vi "TEST_ASIC_MAJnADDS_NEW.vi"(0 "Instrument VISA in":T1={"AWG VISA"="generadorpulsos", "Oscilloscope  VISA "="Oscilloscope", "Integration Board IP"="172.16.7.43", "connection ID"=refnum, "report out"=refnum, "report file path"=path "C:/Documents and Settings/CTA_LAB01/Desktop/L0_Asic/L0 Asic Test Data"}, 1 "threshold":i32[][](array[numeric])=[[518, 513, 533, 498, 543, 508, 548], [526, 521, 546, 506, 551, 516, 556], [534, 529, 549, 514, 559, 524, 564], [542, 537, 557, 522, 567, 532, 572], [545, 540, 565, 530, 575, 530, 575]], 2 "Serial number":string="SN_023", 11 "error in":errorcluster, 13 "Voltages comprobation":dbl[](array[numeric])=[0.05, 0.1, 0.2, 0.5, 0.8]) -> (4 "Instrument VISA out":T1={"AWG VISA"="generadorpulsos", "Oscilloscope  VISA "="Oscilloscope", "Integration Board IP"="172.16.7.43", "connection ID"=refnum, "report out"=refnum, "report file path"=path "C:/Documents and Settings/CTA_LAB01/Desktop/L0_Asic/L0 Asic Test Data"}, 15 "error out":errorcluster)   [LabVIEW 2012]
uses:
  <vilib>/Utility/NIReport.llb/NI_report.lvclass
  Sum_Abrilader/L0_Sum_Adder Folder/C/Program Files/National Instruments/LabVIEW 2012/instr.lib/Agilent 81150/Agilent 81150.lvlib
  <instrlib>/Agilent 8000 Series/Agilent 8000 Series.lvlib
panel:
  in  "Attenuation":i32=15
  in  "NChannels":i32[](array[numeric])=[2, 2, 2, 2, 3, 3, 3, 4, 4, 5, 5, 6, 6, 7]
  in  "Channels Combinations":i32[](array[numeric])=[3, 12, 48, 96, 7, 28, 112, 15, 120, 31, 124, 63, 126, 127]
  out "read buffer 4":string="-1.1741E-08;2.232E-09;9.99999E+37;2.976E-09;3.8996E-01;3.7534E-01\n"
  out "ouput data array":dbl[](array[numeric])=[0.2, 127.0, 0.0, 564.0, 0.0, 0.7653, 0.0, 2.976e-09, 0.0, 9.99999e+37, 0.0, 2.232e-09, 0.0, -1.1741e-08, 0.0, 0.0]
  out "read buffer 3":string="V amptd(f2),1.074E+00,0,1.056E+00,1.087E+00,1.0690E+00,5.5E-03,9.4E+01,+ width(f2),2.90015E-09,0,2.90015E-09,2.95960E-09,2.925838E-09,1.2702E-11,9.4E+01,V amptd(1),5.5E-02,0,4.8E-02,6.7E-02,5.55E-02,3.5E-03,9.4E+01,+ width(f1),9.99999E+37,5,9.99999E+37,9.99999E+37,9.99999E+37,9.99999E+37,9.99999E+37,Time(f1-f2),6.26722E-09,0,6.20145E-09,6.35270E-09,6.264189E-09,3.2805E-11,9.4E+01\n"
  in  "Input Voltages":dbl[](array[numeric])=[0.05, 0.2]
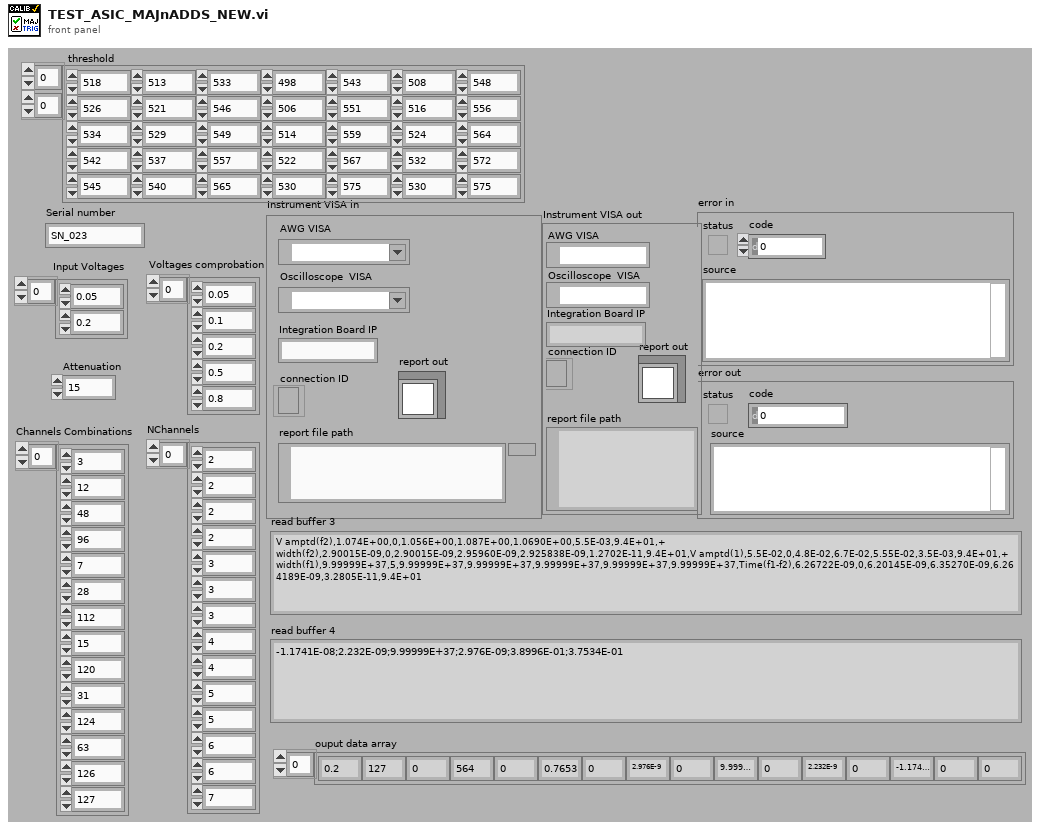
[diagram p1: front panel]
types:
  T1 = cluster{"AWG VISA":refnum<visa-resource-name>, "Oscilloscope  VISA ":refnum<visa-resource-name>, "Integration Board IP":string, "connection ID":refnum<k5>, "report out":refnum<class "NI_report.lvclass">, "report file path":path}
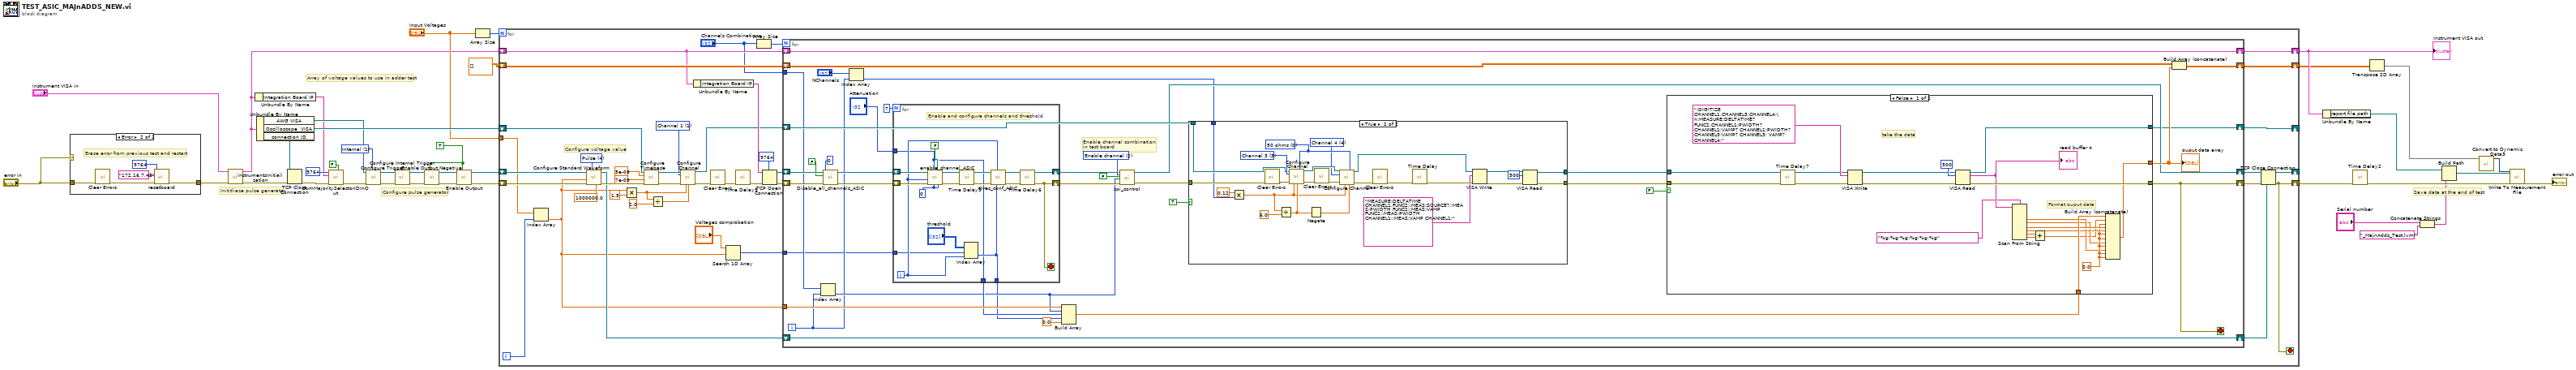
[diagram p0: block diagram]
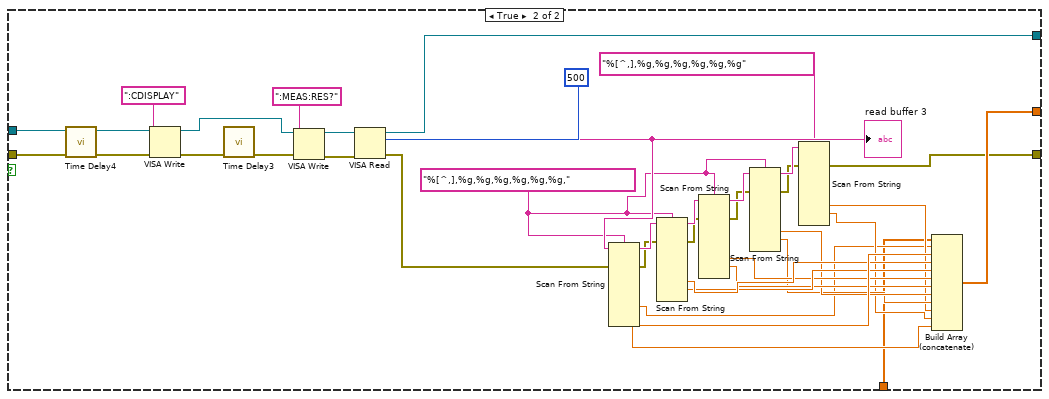
[diagram p3: hidden frame]
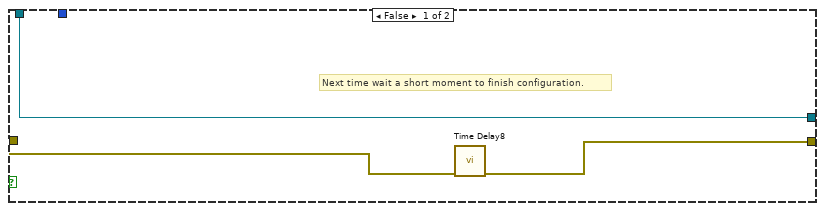
[diagram p4: hidden frame]
diagram:
  w24 = u16 1 items=["Immediate", "Internal", "External", "Software Trigger Function"] ("Trigger Source (0: Immediate)")
  w13 = TRUE ("Enable Output (T: Enable)")
  # "Save data at the end of test"
  # "Array of voltage values to use in adder test"
  # "Configure pulse generator"
  # "Inititliaze pulse generator"
  n1 = case shown="Error" "error in" {
    tunnel: "error in" -> [w39 w41]
    tunnel: [w39 w44] -> w21
    frame No Error {
    }
    frame Error {
      # "Erase error from previous test and restart"
      n2 = call <vilib>:"Clear Errors.vi"("error in (no error)"=w41) -> ("error out"=w40:errorcluster)  [unwired: 6 in]
      n3 = call "resetboard.vi"("error in (no error)"=w40, "address"="172.16.7.43", "remote port or service name"=u16 9764) -> ("error out"=w44:errorcluster)  [unwired: 7 in, 1 out]
    }
  }
  n4 = call "instrumentsInitialization.vi"("error in"=w21, "Instrument VISA in"="Instrument VISA in") -> ("error out"=w19:errorcluster, "Instrument VISA out"=w8:T1)  [unwired: 8 in]
  n5 = Unbundle By Name(w8) -> ("Integration Board IP"=w3:string)
  n6 = Unbundle By Name(w8) -> ("AWG VISA"=w27:refnum<visa-resource-name>, "Oscilloscope  VISA"=w33:refnum<visa-resource-name>, "connection ID"=w20:refnum<k5>)
  n7 = TCP Close Connection(connection ID=w20, error in (no error)=w19) -> (error out=w7:errorcluster)  [unwired: 1 in, 1 out]
  n8 = call "SumMajoritySelectorIDInOut.vi"("On Sum\nOff Majority"=FALSE ("Enable Output (T: Enable)"), "error in"=w7, "address"=w3, "remote port or service name"=u16 9764) -> ("error out"=w6:errorcluster)  [unwired: 7 in]
  n9 = call <instrlib>:"Configure Trigger.vi"("Trigger Source (0: Immediate)"=w24, "error in (no error)"=w6, "VISA resource name"=w27) -> ("error out"=w25:errorcluster, "VISA resource name out"=w26:refnum<visa-resource-name>)  [unwired: 7 in]
  n10 = call <instrlib>:"Configure Internal Trigger.vi"("error in (no error)"=w25, "VISA resource name"=w26) -> ("error out"=w15:errorcluster, "VISA resource name out"=w16:refnum<visa-resource-name>)  [unwired: 8 in]
  n11 = call "Enable Output Negative.vi"("Enable Output (T: Enable)"=w13, "error in (no error)"=w15, "VISA resource name"=w16) -> ("error out"=w14:errorcluster, "VISA resource name out"=w17:refnum<visa-resource-name>)  [unwired: 7 in]
  n12 = call <instrlib>:"Enable Output.vi"("Enable Output (T: Enable)"=w13, "error in (no error)"=w14, "VISA resource name"=w17) -> ("error out"=w2:errorcluster, "VISA resource name out"=w38:refnum<visa-resource-name>)  [unwired: 7 in]
  n13 = Array Size(array="Input Voltages") -> (size(s)=w34:i32)
  n14 = for {
    N: w34 -> [_]
    shift-right: [w75] -> w28
    shift-left: w2 -> [w84]
    tunnel: "Input Voltages" -> [w82]
    shift-right: [w79] -> w18
    shift-left: w8 -> [w52]
    shift-right: [w78] -> w12
    shift-left: dbl[][] [] -> [w80]
    shift-right: [w76] -> _
    shift-left: w38 -> [w83]
    shift-right: [w77] -> _
    shift-left: w33 -> [w81]
    i -> [w46]
    stop <- w75 stop-if-true
    w66 = 1 items=["Channel 1"=1, "Channel 2"=2, "Channel 3"=3, "Channel 4"=4] ("Channel (1: Channel 1)")
    w74 = u16 4 items=["Sine", "Square", "Ramp Up", "Ramp Down", "Pulse", "Noise", "DC"] ("Waveform (0: Sine)")
    # "Configure voltage value"
    n15 = Index Array(array=w82, index=w46) -> (element=w47:dbl)
    n16 = call <instrlib>:"Configure Standard Waveform.vi"("Frequency (1000.0 Hz)"=1000000.0, "Waveform (0: Sine)"=w74, "error in (no error)"=w84, "Amplitude (1.0 Vpp)"=w47, "VISA resource name"=w83) -> ("error out"=w72:errorcluster, "VISA resource name out"=w55:refnum<visa-resource-name>)  [unwired: 5 in]
    n17 = Multiply(x=w47, y=1.5) -> (x*y=w50:dbl)
    n18 = call <instrlib>:"Configure Timebase.vi"("error in (no error)"=w72, "Position (0.0 s)"=7e-09, "Timebase (0.005 s)"=5e-08, "VISA resource name"=w81) -> ("error out"=w71:errorcluster, "VISA resource name out"=w69:refnum<visa-resource-name>)  [unwired: 6 in]
    n19 = Divide(x=w50, y=2.0) -> (x/y=w60:dbl)
    n20 = call <instrlib>:"Configure Channel.vi"("VISA resource name"=w69, "Channel (1: Channel 1)"=w66, "error in (no error)"=w71, "Vertical Range (2.0 V)"=w50, "Vertical Offset (0.0 V)"=w60) -> ("VISA resource name out"=w59:refnum<visa-resource-name>, "error out"=w70:errorcluster)  [unwired: 9 in]
    n21 = Unbundle By Name(w52) -> ("Integration Board IP"=w63:string)
    n22 = call <vilib>:"Clear Errors.vi"("error in (no error)"=w70) -> ("error out"=w54:errorcluster)  [unwired: 6 in]
    n23 = Search 1D Array(1D array="Voltages comprobation", element=w47) -> (index of element=w45:i32)  [unwired: 1 in]
    n24 = call "Time Delay5"("error in (no error)"=w54) -> ("error out"=w53:errorcluster)  [unwired: 10 in]
    n25 = Array Size(array="Channels Combinations") -> (size(s)=w49:i32)
    n26 = TCP Open Connection(address=w63, remote port or service name=u16 9764, error in (no error)=w53) -> (connection ID=w56:refnum<k5>, error out=w64:errorcluster)  [unwired: 2 in]
    n27 = for {
      N: w49 -> [_]
      shift-right: [w106] -> w58
      shift-left: w64 -> [w116]
      shift-right: [w117] -> w78
      shift-left: w80 -> [w118]
      shift-right: [w107] -> w57
      shift-left: w56 -> [w105]
      tunnel: w47 -> [w104]
      shift-right: [w101] -> w77
      shift-left: w59 -> [w110]
      shift-right: [w100] -> w76
      shift-left: w55 -> [w100]
      shift-right: [w96] -> w79
      shift-left: w52 -> [w96]
      tunnel: "Channels Combinations" -> [w93]
      tunnel: w45 -> [w86]
      i -> [w89]
      stop <- w106 stop-if-true
      w115 = u16 2 items=["Attenuation", "Clipping", "Enable channel", "Delay line", "ASIC"] ("Device")
      # "Enable channel combination \nin test board"
      n28 = Index Array(array=w93, index=w89) -> (element=w92:i32)
      n29 = call "Disable_all_channels_ASIC.vi"("error in"=w116, "id_in"=0 ("Data"), "Clip_en_b"=FALSE, "connection ID"=w105) -> ("error out"=w120:errorcluster, "connection ID out"=w119:refnum<k5>)  [unwired: 5 in, 1 out]
      n30 = Index Array(array="NChannels", index=w89) -> (element=w88:i32)
      n31 = for {
        N: u32 7 ("Att gain") -> [_]
        shift-right: [w217] -> w113
        shift-left: w120 -> [w223]
        shift-right: [w218] -> w112
        shift-left: w119 -> [w222]
        tunnel: [w209] -> w103
        tunnel: [w212] -> w91
        tunnel: w86 -> [w210]
        tunnel: "Attenuation" -> [w209]
        i -> [w211]
        stop <- w217 stop-if-true
        w220 = u32 0 ("Ib_clipVb")
        # "Enable and configure channels and threshold"
        n32 = call "enable_channel_ASIC.vi"("Clip_sel_b"=w220, "maj/sum"=FALSE, "Ib_clipVb"=w220, "Att gain"=w209, "error in"=w223, "Channel"=w211, "connection ID"=w222) -> ("error out"=w214:errorcluster, "connection ID out"=w219:refnum<k5>)  [unwired: 2 in, 1 out]
        n33 = call "Time Delay9"("error in (no error)"=w214) -> ("error out"=w215:errorcluster)  [unwired: 10 in]
        n34 = Index Array(array="threshold", index (row)=w210, index (col)=w211) -> (element=w212:i32)
        n35 = call "thres_conf_ASIC.vi"("threshold"=w212, "Ring"=w211, "error out 3"=w215, "connection ID"=w219) -> ("error out 2"=w216:errorcluster, "connection ID out"=w218:refnum<k5>)  [unwired: 4 in, 2 out]
        n36 = call "Time Delay6"("error in (no error)"=w216) -> ("error out"=w217:errorcluster)  [unwired: 10 in]
      }
      n37 = Build Array(w104, w92, w103, w91, 0.0 ("element")) -> (w102:dbl[])
      n38 = call "spi_control.vi"("connection ID"=w112, "Device"=w115, "Read/#write"=FALSE, "Data"=w92, "error out 3"=w113) -> ("connection ID out"=w107:refnum<k5>, "error out 2"=w111:errorcluster)  [unwired: 7 in, 6 out]
      n39 = case shown="True" TRUE {
        tunnel: [w181 w194] -> w98
        tunnel: w111 -> [w182 w189]
        tunnel: w110 -> [w183 w190]
        tunnel: [w183 w200] -> w109
        tunnel: w88 -> [_ w185]
        frame False {
          # "Next time wait a short moment to finish configuration."
          n40 = call "Time Delay8"("error in (no error)"=w182) -> ("error out"=w181:errorcluster)  [unwired: 10 in]
        }
        frame True {
          w201 = u32 0 items=["50 ohms", "1 Mohms"] ("Input Impedance (1: 1 Mohms)")
          w193 = 3 items=["Channel 1"=1, "Channel 2"=2, "Channel 3"=3, "Channel 4"=4] ("Channel (1: Channel 1)")
          w192 = 4 items=["Channel 1"=1, "Channel 2"=2, "Channel 3"=3, "Channel 4"=4] ("Channel (1: Channel 1)")
          n41 = Multiply(x=0.12 ("y"), y=w185) -> (x*y=w186:dbl)
          n42 = call <vilib>:"Clear Errors.vi"("error in (no error)"=w189) -> ("error out"=w207:errorcluster)  [unwired: 6 in]
          n43 = Divide(x=w186, y=6.0) -> (x/y=w187:dbl)
          n44 = call <instrlib>:"Configure Channel.vi"("VISA resource name"=w190, "Input Impedance (1: 1 Mohms)"=w201, "Channel (1: Channel 1)"=w193, "error in (no error)"=w207, "Vertical Range (2.0 V)"=w186, "Vertical Offset (0.0 V)"=w187) -> ("VISA resource name out"=w205:refnum<visa-resource-name>, "error out"=w208:errorcluster)  [unwired: 8 in]
          n45 = Negate(x=w187) -> (-x=w191:dbl)
          n46 = call <vilib>:"Clear Errors.vi"("error in (no error)"=w208) -> ("error out"=w199:errorcluster)  [unwired: 6 in]
          n47 = call <instrlib>:"Configure Channel.vi"("VISA resource name"=w205, "Input Impedance (1: 1 Mohms)"=w201, "Channel (1: Channel 1)"=w192, "error in (no error)"=w199, "Vertical Range (2.0 V)"=w186, "Vertical Offset (0.0 V)"=w191) -> ("VISA resource name out"=w197:refnum<visa-resource-name>, "error out"=w206:errorcluster)  [unwired: 8 in]
          n48 = call <vilib>:"Clear Errors.vi"("error in (no error)"=w206) -> ("error out"=w198:errorcluster)  [unwired: 6 in]
          n49 = call "Time Delay"("error in (no error)"=w198) -> ("error out"=w196:errorcluster)  [unwired: 10 in]
          n50 = VISA Write(VISA resource name=w197, write buffer="MEASURE:DELTATIME CHANNEL1,FUNC2;:MEAS:SOURCE?;:MEAS:PWIDTH FUNC2;:MEAS:VAMP FUNC2;:MEAS:PWIDTH CHANNEL1;:MEAS:VAMP CHANNEL1;", error in (no error)=w196) -> (VISA resource name out=w204:refnum<visa-resource-name>, error out=w203:errorcluster)  [unwired: 1 out]
          n51 = VISA Read(VISA resource name=w204, byte count=u32 500, error in (no error)=w203) -> (VISA resource name out=w200:refnum<visa-resource-name>, error out=w194:errorcluster)  [unwired: 2 out]
        }
      }
      n52 = case shown="False" FALSE {
        tunnel: w109 -> [w139 w151]
        tunnel: [w134 w149] -> w108
        tunnel: [w137 w148] -> w106
        tunnel: w102 -> [w135 w146]
        tunnel: [w136 w145] -> w101
        tunnel: w98 -> [w138 w143]
        frame False {
          w130 = 0.0 ("output 7")
          # "Format ouput data"
          # "take the data"
          n53 = call "Time Delay7"("error in (no error)"=w138) -> ("error out"=w140:errorcluster)  [unwired: 10 in]
          n54 = VISA Write(VISA resource name=w139, write buffer=":DIGITIZE CHANNEL1,CHANNEL3,CHANNEL4;\n:MEASURE:DELTATIME? FUNC2,CHANNEL1;PWIDTH? CHANNEL1;VAMP? CHANNEL1;PWIDTH? CHANNEL3;VAMP? CHANNEL3; VAMP? CHANNEL4;", error in (no error)=w140) -> (VISA resource name out=w133:refnum<visa-resource-name>, error out=w132:errorcluster)  [unwired: 1 out]
          n55 = VISA Read(VISA resource name=w133, byte count=u32 500, error in (no error)=w132) -> (VISA resource name out=w136:refnum<visa-resource-name>, read buffer=w129:string, error out=w137:errorcluster)  [unwired: 1 out]
          "read buffer 4" <- w129
          n56 = Scan From String(format string="%g;%g;%g;%g;%g;%g", input string=w129) -> (output 1=w127:dbl, output 2=w126:dbl, output 3=w131:dbl, output 4=w125:dbl, output 5=w124:dbl, output 6=w123:dbl)  [unwired: 8 in, 3 out]
          n57 = Add(x=w124, y=w123) -> (x+y=w122:dbl)
          n58 = Build Array (concatenate)(w135, w122, w130, w125, w130, w131, w130, w126, w130, w127, w130, w130) -> (w134:dbl[])
        }
        frame True {
          w169 = "%[^,],%g,%g,%g,%g,%g,%g," ("format string")
          n59 = call "Time Delay4"("error in (no error)"=w143) -> ("error out"=w144:errorcluster)  [unwired: 10 in]
          n60 = VISA Write(VISA resource name=w151, write buffer=":CDISPLAY", error in (no error)=w144) -> (VISA resource name out=w154:refnum<visa-resource-name>, error out=w152:errorcluster)  [unwired: 1 out]
          n61 = call "Time Delay3"("error in (no error)"=w152) -> ("error out"=w175:errorcluster)  [unwired: 10 in]
          n62 = VISA Write(VISA resource name=w154, write buffer=":MEAS:RES?", error in (no error)=w175) -> (VISA resource name out=w180:refnum<visa-resource-name>, error out=w179:errorcluster)  [unwired: 1 out]
          n63 = VISA Read(VISA resource name=w180, byte count=u32 500, error in (no error)=w179) -> (VISA resource name out=w145:refnum<visa-resource-name>, read buffer=w176:string, error out=w159:errorcluster)  [unwired: 1 out]
          "read buffer 3" <- w176
          n64 = Scan From String(format string=w169, input string=w176, error in=w159) -> (remaining string=w173:string, error out=w155:errorcluster, output 5=w147:dbl, output 6=w174:dbl, output 7=w160:dbl)  [unwired: 12 in, 1 out]
          n65 = Scan From String(format string=w169, input string=w173, error in=w155) -> (remaining string=w170:string, error out=w156:errorcluster, output 5=w167:dbl, output 6=w166:dbl)  [unwired: 13 in, 1 out]
          n66 = Scan From String(format string=w169, input string=w170, error in=w156) -> (remaining string=w171:string, error out=w157:errorcluster, output 5=w165:dbl, output 6=w164:dbl)  [unwired: 13 in, 1 out]
          n67 = Scan From String(format string=w169, input string=w171, error in=w157) -> (remaining string=w172:string, error out=w158:errorcluster, output 5=w163:dbl, output 6=w162:dbl)  [unwired: 13 in, 1 out]
          n68 = Scan From String(format string="%[^,],%g,%g,%g,%g,%g,%g", input string=w172, error in=w158) -> (error out=w148:errorcluster, output 5=w150:dbl, output 6=w161:dbl)  [unwired: 13 in, 2 out]
          n69 = Build Array (concatenate)(w146, w147, w174, w167, w166, w165, w164, w163, w162, w150, w161, w160) -> (w149:dbl[])
        }
      }
      "ouput data array" <- w108
      n70 = Build Array (concatenate)(w118, w108) -> (w117:dbl[][])
    }
    n71 = TCP Close Connection(connection ID=w57, error in (no error)=w58) -> (error out=w75:errorcluster)  [unwired: 1 in, 1 out]
  }
  "Instrument VISA out" <- w18
  n72 = Unbundle By Name(w18) -> ("report file path"=w37:path)
  n73 = call "Time Delay2"("error in (no error)"=w28) -> ("error out"=w35:errorcluster)  [unwired: 10 in]
  n74 = Transpose 2D Array(2D array=w12) -> (transposed array=w22:dbl[][])
  n75 = Concatenate Strings("Serial number", "_MajnAdds_Test.lvm" ("string")) -> (w11:string)
  n76 = Build Path(base path=w37, name or relative path=w11) -> (appended path=w36:path)
  n77 = call "Convert to Dynamic Data3"("2D Array"=w22) -> ("Dynamic Data Type"=w23:dynamicdata)  [unwired: 3 in]
  n78 = call "Write To Measurement File"("Signals"=w23, "error in (no error)"=w35, "Filename"=w36) -> ("error out"=→"error out":errorcluster)  [unwired: 14 in, 2 out]
